vi "Register Feed.vi"(8 "error in":errorcluster, 10 "feed name":string, 11 "feed URI":string) -> (0 "error out":errorcluster, 2 "registered feed":T1)   [LabVIEW 2014, in "NIPM_API.lvlib"]
doc: "Registers a feed on NI Package Manager on this computer\n\nINPUT(s)\n<b>Feed URI:</b> Specifies the location of the feed (e.g. network folder, web server, etc) to register\n\n<b>Feed name:</b> Specifies the name of the feed to register. If this input is left unwired or empty, NI Package Manager will automatically create a feed name based on the feed URI\n\nOUTPUT(s)\n<b>Registered feed:</b> Outputs the registered feed name and URI, if this VI runs successfully."
uses:
  NIPM_API.lvlib
  _support/feed.ctl
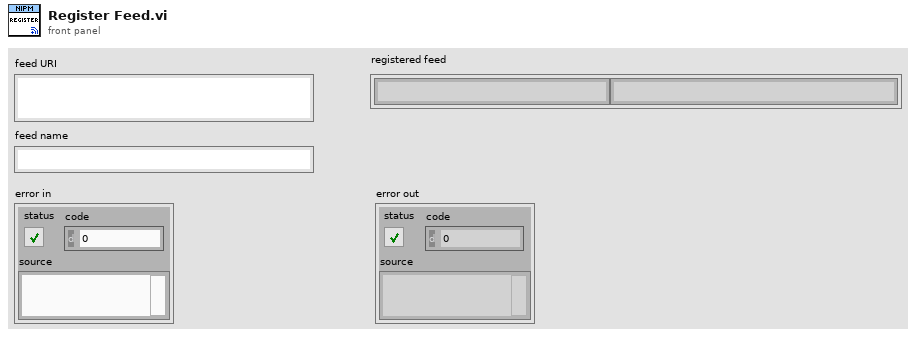
[diagram p1: front panel]
types:
  T1 = typedef "NIPM_API.lvlib/feed.ctl" = cluster{"Name":string, "URI":string}
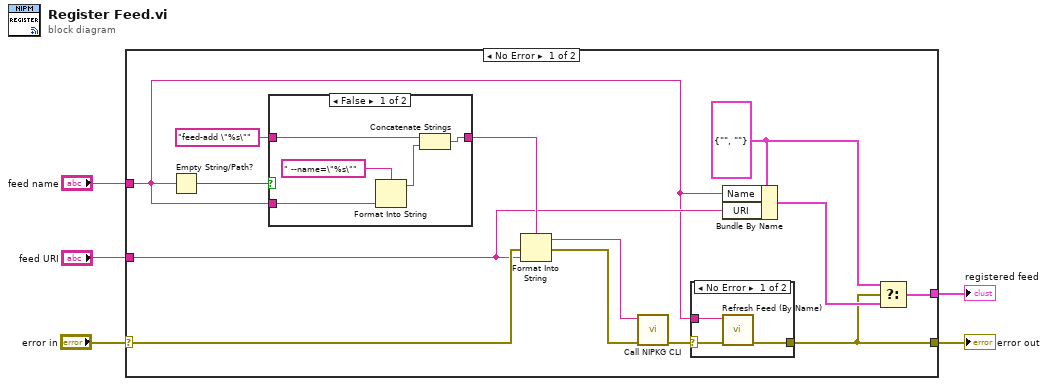
[diagram p0: block diagram]
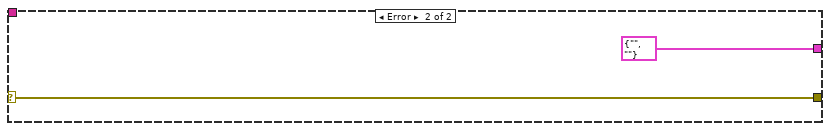
[diagram p4: hidden frame]
diagram:
  n1 = case shown="No Error" "error in" {
    selector: "error in" -> [w18 w30]
    tunnel: [w8 w30] -> w4
    tunnel: "feed URI" -> [w11 _]
    tunnel: "feed name" -> [w7 _]
    tunnel: [w9 T1 {"Name"="", "URI"=""} ("registered feed 2")] -> w1
    frame No Error {
      w13 = T1 {"Name"="", "URI"=""} ("registered feed 2")
      n2 = Empty String/Path?(string/path=w7) -> (empty?=w15:bool)
      n3 = case shown="False" w15 {
        tunnel: w7 -> [w27 _]
        tunnel: "feed-add \"%s\"" ("format string") -> [w25 w28]
        tunnel: [w23 w28] -> w12
        frame False {
          n4 = Format Into String(format string=" --name=\"%s\"", w27) -> (resulting string=w24:string)  [unwired: 2 in, 1 out]
          n5 = Concatenate Strings(w25, w24) -> (w23:string)
        }
        frame True {
        }
      }
      n6 = Format Into String(format string=w12, error in=w18, w11) -> (resulting string=w17:string, error out=w16:errorcluster)  [unwired: 1 in]
      n7 = call "Call NIPKG CLI.vi"("error in (no error)"=w16, "command"=w17) -> ("error out"=w6:errorcluster)  [unwired: 8 in, 1 out]
      n8 = case shown="No Error" w6 {
        selector: w6 -> [w19 w22]
        tunnel: [w21 w22] -> w8
        tunnel: w7 -> [w20 _]
        frame No Error {
          n9 = call "Refresh Feed (By Name).vi"("error in"=w19, "feed name in"=w20) -> ("error out"=w21:errorcluster)  [unwired: 8 in, 1 out]
        }
        frame Error {
        }
      }
      n10 = Bundle By Name(cluster=w13, "Name"=w7, "URI"=w11) -> (w10:T1)
      n11 = Select(t=w13, s=w8, f=w10) -> (s? t:f=w9:T1)
    }
    frame Error {
    }
  }
  "error out" <- w4
  "registered feed" <- w1
